vi "Recta_SubVI.vi"(6 "X1":dbl, 9 "X2":dbl, 10 "Y1":dbl, 11 "Y2":dbl) -> (2 "n":dbl, 3 "m":dbl)   [LabVIEW 2019]
doc: "Calcula el pendent (m) i l'ordenada a l'origen d'una recta donats dos punts (x1, y1), (x2, y2)."
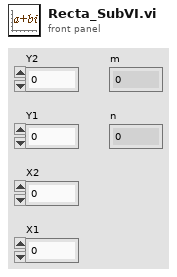
[diagram p1: front panel]
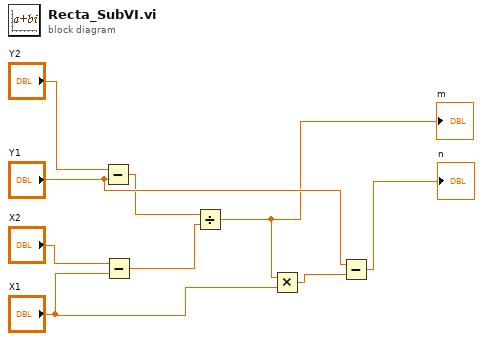
[diagram p0: block diagram]
diagram:
  n1 = Subtract(x="Y2", y="Y1") -> (x-y=w3:dbl)
  n2 = Subtract(x="X2", y="X1") -> (x-y=w4:dbl)
  n3 = Divide(x=w3, y=w4) -> (x/y=w5:dbl)
  "m" <- w5
  n4 = Multiply(x=w5, y="X1") -> (x*y=w7:dbl)
  n5 = Subtract(x="Y1", y=w7) -> (x-y=→"n":dbl)
